vi "CSDB_Common.multilistclick.vi"(2 "Coords":cluster{"Horizontal":i32, "Vertical":i32}, 3 "Multicolumn ref":refnum<vi>) -> (0 "header":string, 1 "coloumn":i32)   [LabVIEW 2014, in "CSDB_Common.lvlib"]
uses:
  CSDB_Common.lvlib
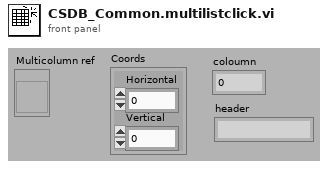
[diagram p1: front panel]
types:
  T1 = typedef "LVPositionTypeDef.ctl" = cluster{"Left":i32, "Top":i32}
  T2 = typedef "LVRowAndColumnTypeDef.ctl" = cluster{"Row":i32, "Column":i32}
  T3 = typedef "LVRowAndColumnUnsignedTypeDef.ctl" = cluster{"Row":u32, "Column":u32}
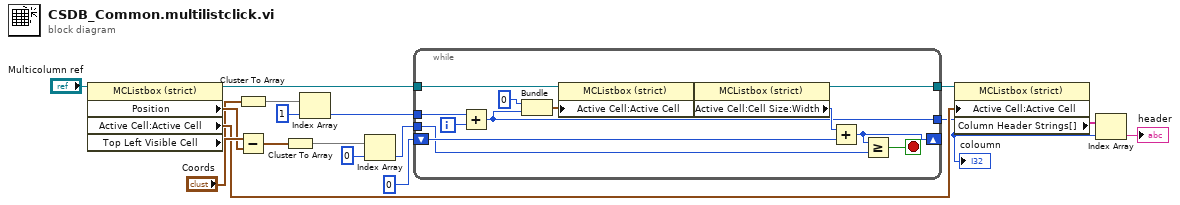
[diagram p0: block diagram]
diagram:
  n1 = property class="MCListbox (strict)"(reference="Multicolumn ref") -> (reference out=w15:refnum<vi>, "Position"=w16:T1, "Active Cell:Active Cell"=w8:T2, "Top Left Visible Cell"=w4:T3)  [unwired: 1 in, 1 out]
  n2 = Cluster To Array(cluster=w4) -> (array=w2:u32[])
  n3 = Subtract(x="Coords", y=w16) -> (x-y=w14:T1)
  n4 = Cluster To Array(cluster=w14) -> (array=w13:i32[])
  n5 = Index Array(array=w2, index=1) -> (element=w1:u32)
  n6 = Index Array(array=w13, index=0) -> (element=w11:i32)
  n7 = while {
    tunnel: w15 -> [w31]
    shift-right: [w25] -> _
    shift-left: u32 0 -> [w26]
    tunnel: w11 -> [w24]
    tunnel: [w19] -> w6
    tunnel: [w22] -> w9
    tunnel: w1 -> [w21]
    i -> [w20]
    stop <- w23 stop-if-true
    n8 = Add(x=w21, y=w20) -> (x+y=w19:u32)
    n9 = Bundle(0, w19) -> (w30:cluster{i32, u32})  [unwired: 1 in]
    n10 = property class="MCListbox (strict)"(reference=w31, "Active Cell:Active Cell"=w30) -> (reference out=w28:refnum<vi>)  [unwired: 1 in, 1 out]
    n11 = property class="MCListbox (strict)"(reference=w28) -> (reference out=w22:refnum<vi>, "Active Cell:Cell Size:Width"=w27:u32)  [unwired: 1 in, 1 out]
    n12 = Add(x=w27, y=w26) -> (x+y=w25:u32)
    n13 = Greater Or Equal?(x=w25, y=w24) -> (x >= y?=w23:bool)
  }
  "coloumn" <- w6
  n14 = property class="MCListbox (strict)"(reference=w9, "Active Cell:Active Cell"=w8) -> ("Column Header Strings[]"=w7:string[])  [unwired: 1 in, 2 out]
  n15 = Index Array(array=w7, index=w6) -> (element=→"header":string)
